vi "ma_One-sided Power Spectrum (CDB).vi"(8 "error in":errorcluster, 10 "dt":dbl format="%0.2f", 11 "signal (V)":cdb[](array[numeric]) format="%0.2f") -> (0 "error out":errorcluster, 2 "df":dbl format="%0.2f", 3 "power spectrum (V^2 rms)":dbl[](array[numeric]) format="%0.2f")   [LabVIEW 2020, in "NI_MAPro.lvlib"]
uses:
  NI_MAPro.lvlib
  NI_AALPro.lvlib
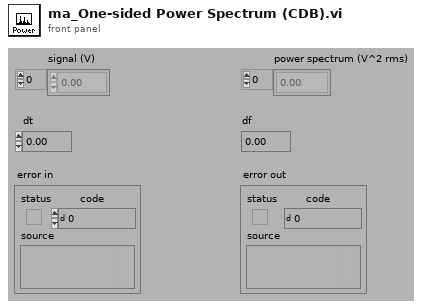
[diagram p1: front panel]
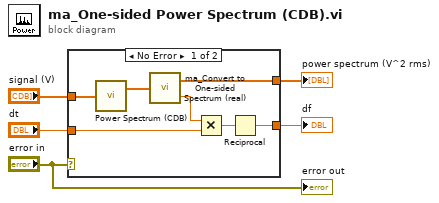
[diagram p0: block diagram]
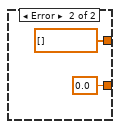
[diagram p2: hidden frame]
diagram:
  n1 = case shown="No Error" "error in" {
    tunnel: "dt" -> [w9 _]
    tunnel: "signal (V)" -> [w8 _]
    tunnel: [w7 0.0] -> w3
    tunnel: [w6 dbl[] [] ("one-sided spectrum (real)")] -> w2
    frame No Error {
      n2 = call "Power Spectrum (CDB).vi"("X"=w8) -> ("Power Spectrum"=w12:dbl[])  [unwired: 1 out]
      n3 = call "ma_Convert to One-sided Spectrum (real).vi"("two-sided spectrum (real)"=w12) -> ("one-sided spectrum (real)"=w6:dbl[], "block size"=w11:dbl)
      n4 = Multiply(x=w11, y=w9) -> (x*y=w10:dbl)
      n5 = Reciprocal(x=w10) -> (1/x=w7:dbl)
    }
    frame Error {
    }
  }
  "power spectrum (V^2 rms)" <- w2
  "df" <- w3
  "error out" <- "error in"
